vi "_dialog_EEPROM_vna_wmg.vi"() -> ()   [LabVIEW 2011]
panel:
  in  "选择sheet":dbl
  in  "路径":path
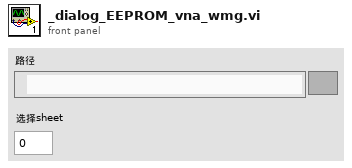
[diagram p1: front panel]
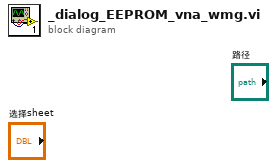
[diagram p0: block diagram]
diagram:
